vi "SMTP Email ConvertToJISB64.vi"(11 "data in":string) -> (3 "data out":string)   [LabVIEW 2011, in "NewNI_SMTPEmail.lvlib"]
doc: "This VI converts an email header field to JIS in Base64 for ISO-2022-JP encoding (RFC 1468)."
uses:
  NewNI_SMTPEmail.lvlib
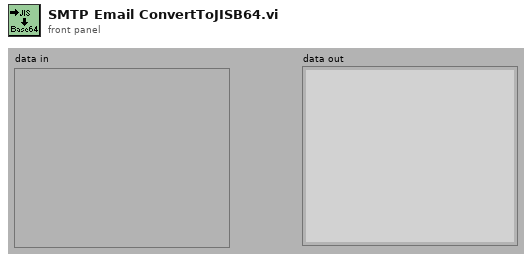
[diagram p1: front panel]
types:
  T1 = enum16{"NOTSET", "NEW", "OLD", "NEC", "EUC", "SJIS", "EUCORSJIS", "ASCII"}
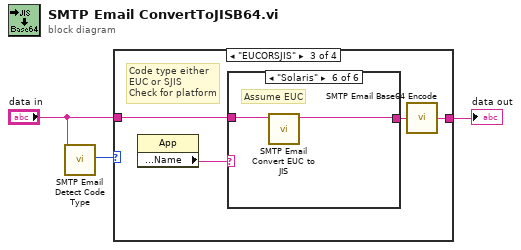
[diagram p0: block diagram]
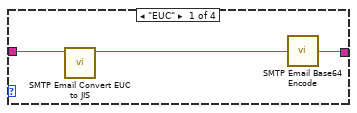
[diagram p2: hidden frame]
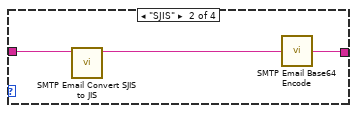
[diagram p3: hidden frame]
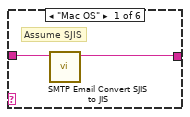
[diagram p4: hidden frame]
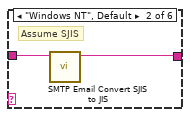
[diagram p5: hidden frame]
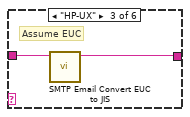
[diagram p6: hidden frame]
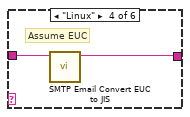
[diagram p7: hidden frame]
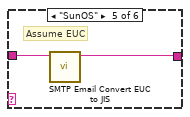
[diagram p8: hidden frame]
diagram:
  n1 = call "SMTP Email Detect Code Type.vi"("text in"="data in") -> ("code type"=w3:T1)  [unwired: 10 out]
  n2 = case shown="\"EUCORSJIS\"" w3 {
    tunnel: "data in" -> [w6 w9 w12 w26]
    tunnel: [w4 w7 w10 w26] -> w1
    frame "EUC" {
      n3 = call "SMTP Email Convert EUC to JIS.vi"("text in"=w6) -> ("text out"=w5:string)  [unwired: 10 out]
      n4 = call "SMTP Email Base64 Encode.vi"("Normal String"=w5) -> ("Base64 String"=w4:string)  [unwired: 1 in]
    }
    frame "SJIS" {
      n5 = call "SMTP Email Convert SJIS to JIS.vi"("text in"=w9) -> ("text out"=w8:string)  [unwired: 1 in, 9 out]
      n6 = call "SMTP Email Base64 Encode.vi"("Normal String"=w8) -> ("Base64 String"=w7:string)  [unwired: 1 in]
    }
    frame "EUCORSJIS" {
      # "Code type either \nEUC or SJIS\nCheck for platform"
      n7 = property class="App"() -> ("Operating System:Name"=w13:string)  [unwired: 2 in, 2 out]
      n8 = case shown="\"Solaris\"" w13 {
        tunnel: w12 -> [w15 w17 w19 w21 w23 w25]
        tunnel: [w14 w16 w18 w20 w22 w24] -> w11
        frame "Mac OS" {
          # "Assume SJIS"
          n9 = call "SMTP Email Convert SJIS to JIS.vi"("text in"=w15) -> ("text out"=w14:string)  [unwired: 1 in, 9 out]
        }
        frame "Windows NT", Default {
          # "Assume SJIS"
          n10 = call "SMTP Email Convert SJIS to JIS.vi"("text in"=w17) -> ("text out"=w16:string)  [unwired: 1 in, 9 out]
        }
        frame "HP-UX" {
          # "Assume EUC"
          n11 = call "SMTP Email Convert EUC to JIS.vi"("text in"=w19) -> ("text out"=w18:string)  [unwired: 10 out]
        }
        frame "Linux" {
          # "Assume EUC"
          n12 = call "SMTP Email Convert EUC to JIS.vi"("text in"=w21) -> ("text out"=w20:string)  [unwired: 10 out]
        }
        frame "SunOS" {
          # "Assume EUC"
          n13 = call "SMTP Email Convert EUC to JIS.vi"("text in"=w23) -> ("text out"=w22:string)  [unwired: 10 out]
        }
        frame "Solaris" {
          # "Assume EUC"
          n14 = call "SMTP Email Convert EUC to JIS.vi"("text in"=w25) -> ("text out"=w24:string)  [unwired: 10 out]
        }
      }
      n15 = call "SMTP Email Base64 Encode.vi"("Normal String"=w11) -> ("Base64 String"=w10:string)  [unwired: 1 in]
    }
    frame "ASCII", Default {
      # "If code type is not of type\nSJIS or EUC, then do nothing"
    }
  }
  "data out" <- w1
